vi "Goal Vision Align.vi"(11 "Goal Vision Packet":T1) -> (2 "Aligned?":bool, 3 "Turn Power":dbl)   [LabVIEW 2015]
uses:
  Common Code/Goal Vision Packet.ctl
  Robot Global Data.vi
  <vilib>/addons/control/pid/pid.llb/PID (DBL).vi
  <vilib>/addons/control/pid/NI_PID_pid.lvlib
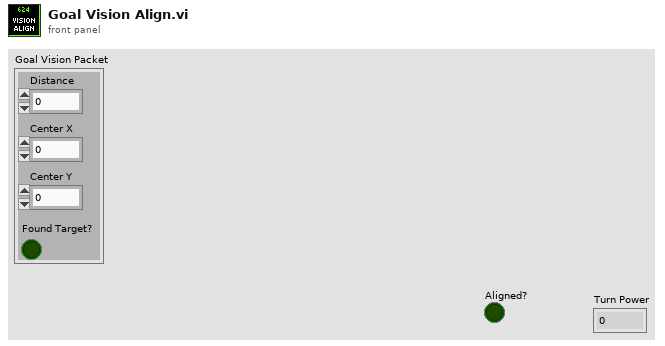
[diagram p1: front panel]
types:
  T1 = typedef "Goal Vision Packet.ctl" = cluster{"Distance":dbl, "Center X":dbl, "Center Y":dbl, "Found Target?":bool}
  T2 = typedef "Dashboard Control Data.ctl" = cluster{"Shooter Presets":T3, "Encoder Control":T5, "Steer PID output":cluster{"output high":dbl, "output low":dbl}, " Steer PID gains":cluster{"proportional gain (Kc)":dbl, "integral time (Ti, min)":dbl, "derivative time (Td, min)":dbl}, "Drivetrain Settings":T6, "Vision Packet":T1, "Dashboard Drivetrain Command":T7, "Info/Command Cluster":T9, "Ball Vision Packet":T10, "Intake Presets":T12, "Intake Encoder Control":T14, "Climb Presets":T15, "Goal Output Range":cluster{"output high":dbl, "output low":dbl}}
  T3 = typedef "Shooter Presets.ctl" = cluster{"Batter Shot":T4, "Low Bar Curve Shot":T4, "Deep Middle Shot":T4, "Manual Shot":T4, "Left Ticks Per Rotation":dbl, "Right Ticks Per Rotation":dbl, "Low Bar Shot":T4, "Shooter RPM Tolerance":dbl, "IIR Filter Power":dbl, "Trigger Power":dbl, "Fire from Load Delay":i32, "Angle Pot M":dbl, "Angle Pot B":dbl, "Shooter Deck Length":dbl, "String Pot Dist From Pivot":dbl, "Angle PID gains":cluster{"proportional gain (Kc)":dbl, "integral time (Ti, min)":dbl, "derivative time (Td, min)":dbl}, "Angle Motor Output Range":cluster{"output high":dbl, "output low":dbl}, "Shooter Angle Tolerance":dbl, "Vision Shoot x^2":dbl, "Vision Shoot x":dbl, "Dist from Axis Cam to Pivot":dbl, "High Goal Center Height":dbl, "Feed Forward Max Accel":dbl, "Feed Forward Kv":dbl, "Backwards Trigger":dbl, "Shot Finish Delay (ms)":dbl, "Angle Max Current":dbl, "Angle Current Trip Time":dbl, "Shooter Intake Angle":dbl, "Vision Shoot c":dbl}
  T4 = typedef "Shot Presets.ctl" = cluster{"Left Wheel RPM":dbl, "Right Wheel RPM":dbl, "Angle":dbl}
  T5 = typedef "Encoder Control.ctl" = cluster{"Right Tick Constant":dbl, "Left Tick Constant":dbl, "Reset?":bool, "Y Dist":cluster{"PID gains":cluster{"proportional gain (Kc)":dbl, "integral time (Ti, min)":dbl, "derivative time (Td, min)":dbl}}, "Y Stop Thresh":dbl, "Y Stop Speed":dbl}
  T6 = typedef "Drivetrain Settings.ctl" = cluster{"Gyro Tolerance":dbl, "Throttle Ramp (ms)":dbl, "Angular rate compensation":bool, "Throttle to Rate Scale":dbl, "Rate compensation gain":dbl, "Kv":dbl, "Ka":dbl, "Feed Forward P":dbl, "Feed Forward D":dbl, "Goal Vision PID gains":cluster{"proportional gain (Kc)":dbl, "integral time (Ti, min)":dbl, "derivative time (Td, min)":dbl}, "Goal Detection Window":dbl}
  T7 = typedef "Dashboard Drivetrain Command.ctl" = cluster{"Drivetrain Vision":T8}
  T8 = typedef "Drivetrain Vision.ctl" = cluster{"Goal Window":dbl, "Ball Window":dbl}
  T9 = typedef "Ball Tracking Command Cluster.ctl" = cluster{"Distance to Ball":dbl, "Desired Angle":dbl, "Command":enum16{"Turn to Ball", "Turn to Angle", "Get Distance"}, "Pixels from Center":dbl}
  T10 = typedef "Ball Vision Packet.ctl" = cluster{"Ball Detected?":bool, "Distance to Ball":dbl, "Desired Angle":dbl, "Pixels from Center":dbl, "Tracking mode":T11}
  T11 = typedef "Tracking Mode.ctl" = enum16{"Turn to Ball", "Turn to Angle"}
  T12 = typedef "Intake Presets.ctl" = cluster{"Intake Speed":dbl, "Outake Speed":dbl, "Low Height":dbl, "Half Height":dbl, "Full Height":dbl, "Angle Speed":dbl, "Fast Angle":dbl, "Encoder Scale Factor":dbl, "Load Height":dbl, "Output Range":T13, "PID Params":cluster{"PID gains":cluster{"proportional gain (Kc)":dbl, "integral time (Ti, min)":dbl, "derivative time (Td, min)":dbl}}, "Rotation Power Max/Min":dbl, "MaxCurrent":dbl, "Intake Trip Time":dbl, "Idle Height":dbl, "Max Height":dbl}
  T13 = typedef "Drivetrain Output Range.ctl" = cluster{"output high":dbl, "output low":dbl}
  T14 = typedef "IntakeEcoderControl.ctl" = cluster{"Arm Tick Constant":dbl, "Reset?":bool, "Y Dist":cluster{"PID gains":cluster{"proportional gain (Kc)":dbl, "integral time (Ti, min)":dbl, "derivative time (Td, min)":dbl}}, "Y Stop Thresh":dbl, "Y Stop Speed":dbl}
  T15 = typedef "Climb Presets.ctl" = cluster{"Pull Power":dbl, "Unpin Power":dbl, "Time to Hold":dbl}
  T16 = cluster{"proportional gain (Kc)":dbl, "integral time (Ti, min)":dbl, "derivative time (Td, min)":dbl}
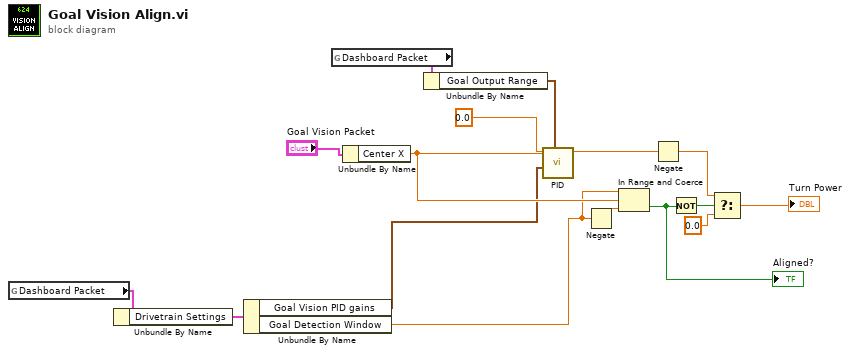
[diagram p0: block diagram]
diagram:
  n1 = global read "Robot Global Data.vi" "Dashboard Packet"() -> (w2:T2)
  n2 = Unbundle By Name(w2) -> ("Drivetrain Settings"=w1:T6)
  n3 = Unbundle By Name(w1) -> ("Goal Vision PID gains"=w7:T16, "Goal Detection Window"=w6:dbl)
  n4 = global read "Robot Global Data.vi" "Dashboard Packet"() -> (w5:T2)
  n5 = Unbundle By Name("Goal Vision Packet") -> ("Center X"=w11:dbl)
  n6 = Unbundle By Name(w5) -> ("Goal Output Range"=w4:cluster{"output high":dbl, "output low":dbl})
  n7 = call-poly <vilib>:"PID.vi"("output range"=w4, "PID gains"=w7, "process variable"=w11, "setpoint"=0.0) -> ("output"=w15:dbl)  [unwired: 6 in, 1 out]
  n8 = Negate(x=w6) -> (-x=w8:dbl)
  n9 = In Range and Coerce(upper limit=w6, x=w11, lower limit=w8) -> (In Range?=w12:bool)  [unwired: 1 out]
  "Aligned?" <- w12
  n10 = Negate(x=w15) -> (-x=w16:dbl)
  n11 = Not(x=w12) -> (.not. x?=w13:bool)
  n12 = Select(t=w16, s=w13, f=0.0 ("t")) -> (s? t:f=→"Turn Power":dbl)
